vi "Get Raw Data and Send To FPGA.vi"(8 "error in (no error)":errorcluster) -> (0 "error out":errorcluster)   [LabVIEW 2017]
doc: "Retrieves samples from the RTL-SDR device and passes them on to the fpga for processing."
uses:
  FPGA Control/FPGA Global Variables.vi
  Utilities/Application Globals.vi
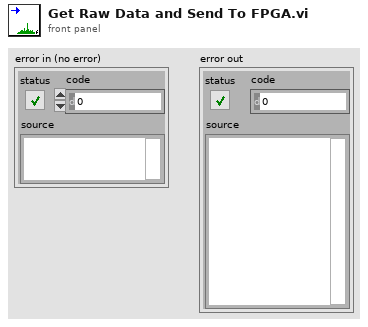
[diagram p1: front panel]
types:
  T1 = typedef "rtltcp_RTLTCP Configuraton.ctl" = cluster{"RTL TCP Connection ID":refnum<k5>, "Center Frequency":u32, "Sample Rate (Bandwith)":u32, "Gain (dB)":dbl, "Frequency Correction (ppm)":i32, "Tuner Auto Gain Mode":bool, "AGC":bool}
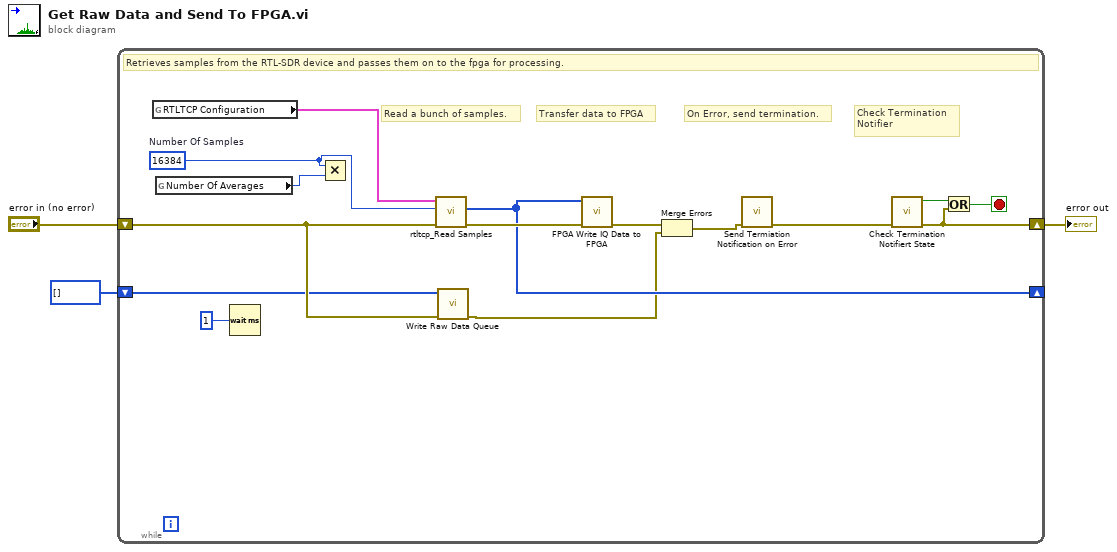
[diagram p0: block diagram]
diagram:
  n1 = while {
    shift-right: [w15] -> w2
    shift-left: "error in (no error)" -> [w12]
    shift-right: [w13] -> _
    shift-left: u8[] [] ("Sample Buffer") -> [w6]
    stop <- w14 stop-if-true
    w7 = 16384  # Number Of Samples
    # "On Error, send termination."
    # "Check Termination\nNotifier"
    # "Transfer data to FPGA"
    # "Read a bunch of samples."
    # "Retrieves samples from the RTL-SDR device and passes them on to the fpga for processing."
    n2 = global read "Application Globals.vi" "RTLTCP Configuration"() -> (w5:T1)
    n3 = global read "FPGA Global Variables.vi" "Number Of Averages"() -> (w9:u32)
    n4 = Wait (ms)(milliseconds to wait=u32 1) -> ()  [unwired: 1 out]
    n5 = Multiply(x=w7, y=w9) -> ()  [unwired: 1 out]
    n6 = call "rtltcp_Read Samples.vi"("error in (no error)"=w12, "Sample Count"=w7, "RTL TCP Configuration In"=w5) -> ("error out"=w17:errorcluster, "Sample Buffer"=w13:u8[])  [unwired: 6 in, 1 out]
    n7 = call "Write Raw Data Queue.vi"("error in (no error)"=w12, "Sample Buffer"=w6) -> ("error out"=w4:errorcluster)  [unwired: 9 in]
    n8 = call "FPGA Write IQ Data to FPGA.vi"("error in (no error)"=w17, "Sample Buffer"=w13) -> ("error out"=w11:errorcluster)  [unwired: 9 in]
    n9 = Merge Errors(w11, w4) -> (w10:errorcluster)
    n10 = call "Send Termiation Notification on Error.vi"("error in (no error)"=w10) -> ("error out"=w18:errorcluster)  [unwired: 10 in]
    n11 = call "Check Termination Notifiert State.vi"("error in (no error)"=w18) -> ("error out"=w15:errorcluster, "Termination Notifier State"=w16:bool)  [unwired: 9 in]
    n12 = Or(x=w16, y=w15) -> (x .or. y?=w14:bool)
  }
  "error out" <- w2
